vi "Simulated Camera.TestLauncher.vi"() -> ()   [LabVIEW 2013]
doc: "JKI State Machine Objects (SMO) 1.0.0.5\nJKI - JKI\nCopyright (c) 2016, JKI"
uses:
  <vilib>/JKI/JKI SMO/SMO/SMO.lvclass
  Camera/Camera.lvclass
  <vilib>/JKI/JKI SMO/SMO/Typedefs/SMOState --Enum.ctl
  <vilib>/Utility/error.llb/DialogType.ctl
  Camera.IMAQdx/Camera.IMAQdx.lvclass
  Camera.Simulated.lvclass
panel:
  in  "Camera Type":enum16{"Simulated", "IMAQdx"}(ring)
  in  "Filepath":path
  in  "Save":bool
  out "Buffer":i32
  out "Image":picture
  out "State":T1
  in  "Grab":bool
  out "error out":errorcluster
  in  "Stop":bool
  # "Camera Test Launcher"
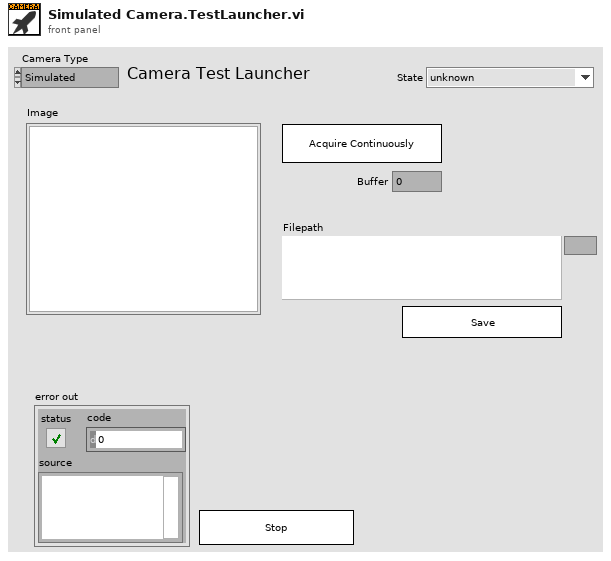
[diagram p1: front panel]
types:
  T1 = typedef "SMO.lvclass/SMOState --Enum.ctl" = enum16{"unknown", "Created", "Started", "Stopped"}
  T2 = typedef "Camera.lvclass/PublicEvents--Cluster.ctl" = cluster{"NewImage":refnum<user-event>, "ImageSaved":refnum<user-event>}
  T3 = typedef "SMO.lvclass/Public Events.ctl" = cluster{"Error":refnum<user-event>, "State":refnum<user-event>}
  T4 = cluster{"Event Registration Refnum":refnum<event-registration>}
  T5 = typedef "DialogType.ctl" = u16
  T6 = typedef "imagedata.ctl" = cluster{"image type":i32, "image depth":i32, "image":u8[], "mask":u8[], "colors":u32[], "Rectangle":cluster{"left":i16, "top":i16, "right":i16, "bottom":i16}}
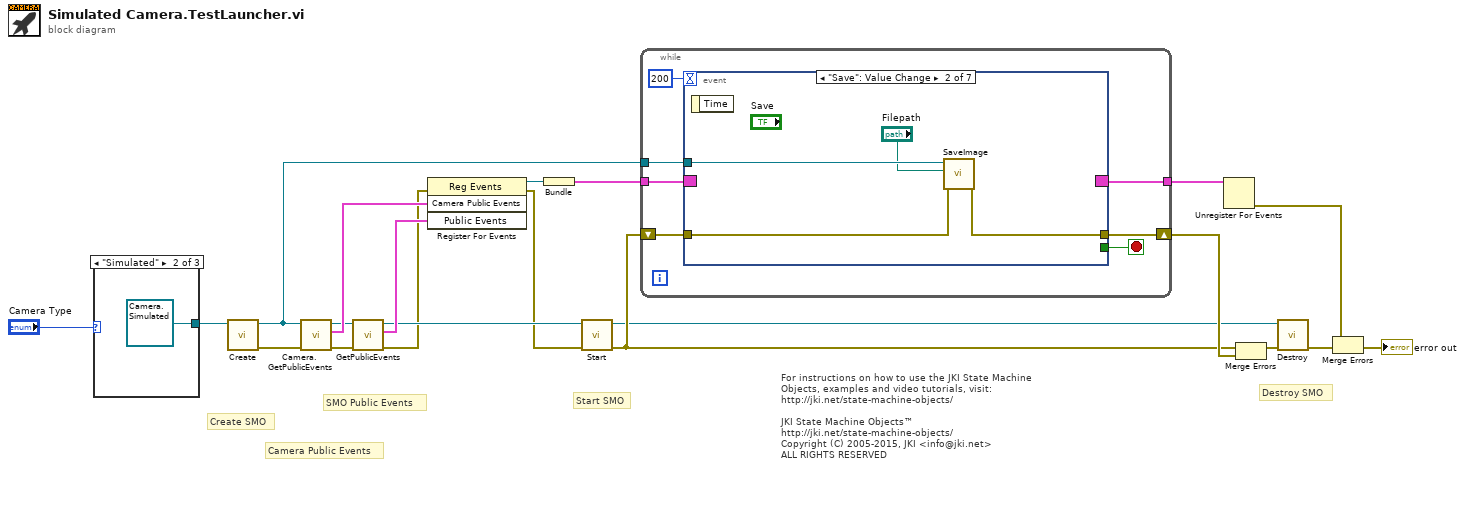
[diagram p0: block diagram]
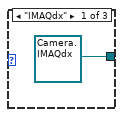
[diagram p2: hidden frame]
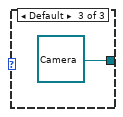
[diagram p3: hidden frame]
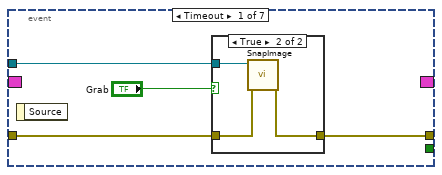
[diagram p4: hidden frame]
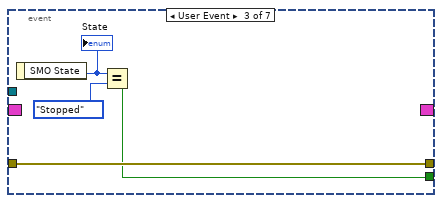
[diagram p6: hidden frame]
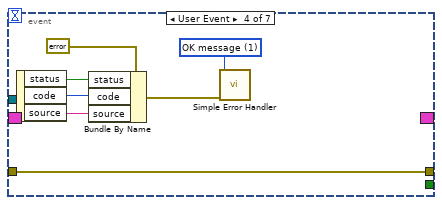
[diagram p7: hidden frame]
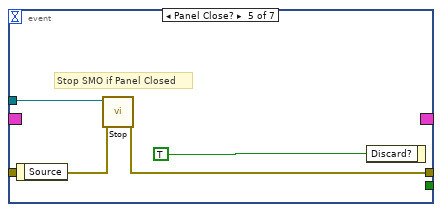
[diagram p8: hidden frame]
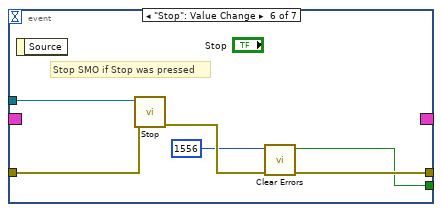
[diagram p9: hidden frame]
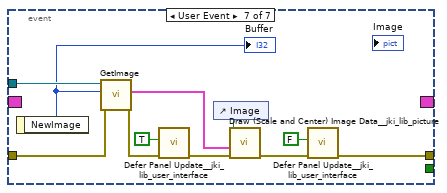
[diagram p10: hidden frame]
diagram:
  # "SMO Public Events"
  # "For instructions on how to use the JKI State Machine Objects, examples and video tutorials, visit:\nhttp://jki.net/state-machine-objects/\n\nJKI State Machine Objects™\nhttp://jki.net/state-machine-objects/\nCopyright (C) 2005-2015, JKI <info@jki.net>\nALL RIGHTS RESERVED"
  # "Camera Public Events"
  # "Start SMO"
  # "Destroy SMO"
  # "Create SMO"
  n1 = case shown="\"Simulated\"" "Camera Type" {
    tunnel: [refnum<class "Camera.IMAQdx.lvclass"> refnum ("Camera.IMAQdx in") refnum<class "Camera.Simulated.lvclass"> refnum ("Camera.Simulated in") refnum<class "Camera.lvclass"> refnum ("SMO.Template.lvclass")] -> w1
    frame "IMAQdx" {
    }
    frame "Simulated" {
    }
    frame Default {
    }
  }
  n2 = call <vilib>:"Create.vi"("SMO"=w1) -> ("error out"=w3:errorcluster, "SMO out"=w2:refnum<class "Camera.lvclass">)  [unwired: 8 in, 1 out]
  n3 = call "Camera.GetPublicEvents.vi"("error in (no error)"=w3, "Camera"=w2) -> ("error out"=w11:errorcluster, "Camera Public Events"=w14:T2, "Camera out"=w12:refnum<class "Camera.lvclass">)  [unwired: 7 in]
  n4 = call <vilib>:"GetPublicEvents.vi"("error in (no error)"=w11, "SMO"=w12) -> ("error out"=w8:errorcluster, "Public Events"=w10:T3, "SMO out"=w9:refnum<class "Camera.lvclass">)  [unwired: 7 in]
  n5 = register-events(error in=w8, w14, w10) -> (reference out=w13:refnum<event-registration>, error out=w7:errorcluster)  [unwired: 1 in]
  n6 = Bundle("Event Registration Refnum"=w13) -> (w20:T4)  [unwired: 1 in]
  n7 = call <vilib>:"Start.vi"("error in (no error)"=w7, "SMO"=w9) -> ("error out"=w15:errorcluster, "SMO out"=w5:refnum<class "Camera.lvclass">)  [unwired: 8 in]
  n8 = while {
    shift-right: [w30] -> w19
    shift-left: w15 -> [w29]
    tunnel: w20 -> [w28]
    tunnel: [w27] -> w21
    tunnel: w2 -> [w26]
    stop <- w31 stop-if-true
    n9 = event shown="[1] \"Save\": Value Change" {
      selector: w28 -> [_ _ _ _ _ _ _]
      dyn-events: [_ _ _ _ _ _ _] -> w27
      timeout: 200 -> [_ _ _ _ _ _ _]
      tunnel: [_ _ w44 _ _ w59 _] -> w31
      tunnel: w26 -> [w35 w43 _ _ w58 w64 w75]
      tunnel: [w33 w41 w47 w54 w57 w61 w65] -> w30
      tunnel: w29 -> [w34 w42 w47 w54 w56 w63 w73]
      event Timeout {
        n10 = event-data() -> ()  [unwired: 1 in, 1 out]
        n11 = case shown="True" "Grab" {
          tunnel: w35 -> [_ w39]
          tunnel: w34 -> [w36 w38]
          tunnel: [w36 w37] -> w33
          frame False {
          }
          frame True {
            n12 = call "SnapImage.vi"("error in (no error)"=w38, "Camera"=w39) -> ("error out"=w37:errorcluster)  [unwired: 7 in, 2 out]
          }
        }
      }
      event "Save": Value Change {
        n13 = event-data() -> ()  [unwired: 1 in, 1 out]
        n14 = call "SaveImage.vi"("error in (no error)"=w42, "Path"="Filepath", "Camera"=w43) -> ("error out"=w41:errorcluster)  [unwired: 7 in, 1 out]
      }
      event User Event {
        n15 = event-data() -> ("SMO State"=w46:T1)  [unwired: 1 in]
        "State" <- w46
        n16 = Equal?(x=w46, y=SMOState_--Enum."Stopped") -> (x = y?=w44:bool)
      }
      event User Event {
        w48 = T5 1 items=["no dialog", "OK message", "continue or stop message", "OK message + warnings", "continue/stop + warnings"] ("type of dialog (OK msg:1)")
        n17 = event-data() -> ("status"=w52:bool, "code"=w51:i32, "source"=w50:string)  [unwired: 1 in]
        n18 = Bundle By Name(cluster=errorcluster {"status"=FALSE, "code"=0, "source"=""} ("error out"), "status"=w52, "code"=w51, "source"=w50) -> (w49:errorcluster)
        n19 = call <vilib>:"Simple Error Handler.vi"("type of dialog (OK msg:1)"=w48, "error in (no error)"=w49) -> ()  [unwired: 3 in, 5 out]
      }
      event Panel Close? {
        # "Stop SMO if Panel Closed"
        n20 = event-data() -> ()  [unwired: 1 in, 1 out]
        n21 = call <vilib>:"Stop.vi"("error in (no error)"=w56, "SMO"=w58) -> ("error out"=w57:errorcluster)  [unwired: 8 in, 1 out]
        n22 = event-data("Discard?"=TRUE ("OK")) -> ()  [unwired: 1 in, 1 out]
      }
      event "Stop": Value Change {
        # "Stop SMO if Stop was pressed"
        n23 = event-data() -> ()  [unwired: 1 in, 1 out]
        n24 = call <vilib>:"Stop.vi"("error in (no error)"=w63, "SMO"=w64) -> ("error out"=w62:errorcluster)  [unwired: 8 in, 1 out]
        n25 = call <vilib>:"Clear Errors.vi"("error in (no error)"=w62, "specific error code to clear (0: all)"=1556) -> ("error out"=w61:errorcluster, "specific error cleared?"=w59:bool)  [unwired: 4 in]
      }
      event User Event {
        n26 = event-data() -> ("NewImage"=w74:i32)  [unwired: 1 in]
        "Buffer" <- w74
        n27 = call "GetImage.vi"("error in (no error)"=w73, "Get Image (-1: latest)"=w74, "Camera"=w75) -> ("error out"=w70:errorcluster, "image data"=w72:T6)  [unwired: 6 in, 1 out]
        n28 = call <vilib>:"Defer Panel Update__jki_lib_user_interface.vi"("error in (no error)"=w70, "defer panel updates"=TRUE) -> ("error out"=w69:errorcluster)  [unwired: 8 in, 1 out]
        n29 = control-ref of="Image"() -> (w71:refnum<vi>)
        n30 = call <vilib>:"Draw (Scale and Center) Image Data__jki_lib_picture.vi"("Error In"=w69, "Image Data In"=w72, "Picture Ref In"=w71) -> ("Error Out"=w66:errorcluster)  [unwired: 7 in, 1 out]
        n31 = call <vilib>:"Defer Panel Update__jki_lib_user_interface.vi"("error in (no error)"=w66, "defer panel updates"=FALSE) -> ("error out"=w65:errorcluster)  [unwired: 8 in, 1 out]
      }
    }
  }
  n32 = Unregister For Events(event registration refnum=w21) -> (error out=w18:errorcluster)  [unwired: 1 in]
  n33 = Merge Errors(w15, w19) -> (w6:errorcluster)
  n34 = call <vilib>:"Destroy.vi"("error in (no error)"=w6, "SMO"=w5) -> ("error out"=w16:errorcluster)  [unwired: 9 in]
  n35 = Merge Errors(w18, w16) -> (→"error out":errorcluster)
